vi "Delete DVR.vi"(0 "Device DVR":refnum<data-value>, 11 "Error in":errorcluster) -> (4 "Device Class Out":refnum<class "Device.lvclass">, 15 "Error out":errorcluster)   [LabVIEW 2020, in "Device.lvclass"]
doc: "Delete DVR reference"
uses:
  Device.lvclass
  Device.lvclass/Device.ctl
panel:
  out "Device out":refnum<class "Device.lvclass">
  in  "Device in":refnum<class "Device.lvclass">
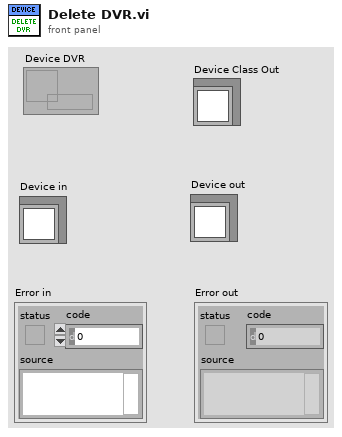
[diagram p1: front panel]
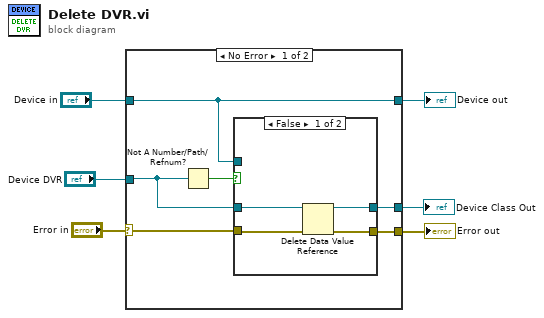
[diagram p0: block diagram]
diagram:
  n1 = case shown="No Error" "Error in" {
    selector: "Error in" -> [w10 w20]
    tunnel: [w9 w20] -> w4
    tunnel: [w7 w19] -> w3
    tunnel: "Device in" -> [w7 w19]
    tunnel: "Device DVR" -> [w11 _]
    tunnel: [w8 w19] -> w1
    frame No Error {
      n2 = Not A Number/Path/Refnum?(number/path/refnum=w11) -> (NaN/Path/Refnum?=w12:bool)
      n3 = case shown="False" w12 {
        tunnel: w11 -> [w15 _]
        tunnel: w10 -> [w16 w18]
        tunnel: [w14 w18] -> w9
        tunnel: [w13 w17] -> w8
        tunnel: w7 -> [_ w17]
        frame False {
          n4 = Delete Data Value Reference(data value reference=w15, error in=w16) -> (data value=w13:refnum<class "Device.lvclass">, error out=w14:errorcluster)
        }
        frame True {
        }
      }
    }
    frame Error {
    }
  }
  "Error out" <- w4
  "Device out" <- w3
  "Device Class Out" <- w1
